vi "Remove Resource.vi"(8 "error in (no error)":errorcluster, 10 "RID":string, 11 "LangFile in":refnum<class "Resource Data.lvclass">) -> (0 "error out":errorcluster, 3 "LangFile out":refnum<class "Resource Data.lvclass">)   [LabVIEW 2013, in "SET Project Data.lvlib" / "Resource Data.lvclass"]
uses:
  Resource Data.lvclass
  Resource Data.lvclass/Resource Data.ctl
  Read Resources.vi
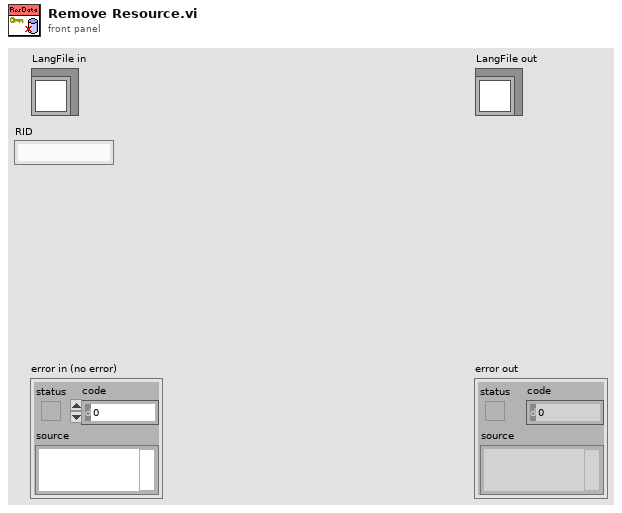
[diagram p1: front panel]
types:
  T1 = typedef "SET Project Data.lvlib/ProjFile_Resource Data.ctl" = cluster{"RID":string, "Tag":string, "Strings [] (UTF-16)":string[], "Shared?":bool}
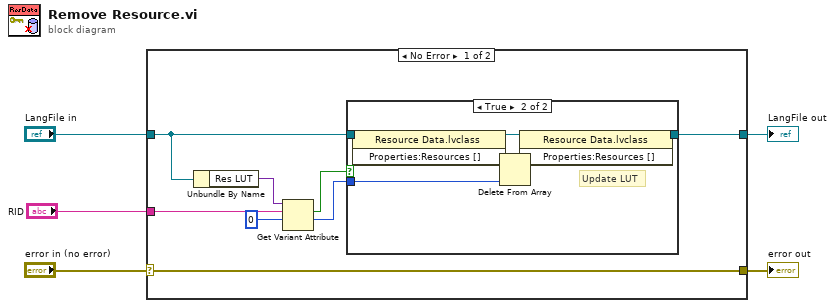
[diagram p0: block diagram]
diagram:
  n1 = case shown="No Error" "error in (no error)" {
    selector: "error in (no error)" -> [w13 w22]
    tunnel: [w13 w22] -> w4
    tunnel: [w6 w21] -> w2
    tunnel: "LangFile in" -> [w7 w21]
    tunnel: "RID" -> [w11 _]
    frame No Error {
      n2 = Unbundle By Name(w7) -> ("Res LUT"=w10:variant)
      n3 = Get Variant Attribute(Variant=w10, name=w11, default value (empty Variant)=0) -> (found=w9:bool, value=w8:i32)  [unwired: 1 in, 2 out]
      n4 = case shown="True" w9 {
        tunnel: w8 -> [_ w20]
        tunnel: w7 -> [w14 w18]
        tunnel: [w14 w19] -> w6
        frame False {
        }
        frame True {
          # "Update LUT"
          n5 = property class="Resource Data.lvclass"(reference=w18) -> (reference out=w15:refnum<class "Resource Data.lvclass">, "Properties:Resources []"=w17:T1[])  [unwired: 1 in, 1 out]
          n6 = Delete From Array(array=w17, index=w20) -> (array with subset deleted=w16:T1[])  [unwired: 1 in, 1 out]
          n7 = property class="Resource Data.lvclass"(reference=w15, "Properties:Resources []"=w16) -> (reference out=w19:refnum<class "Resource Data.lvclass">)  [unwired: 1 in, 1 out]
        }
      }
    }
    frame Error {
    }
  }
  "error out" <- w4
  "LangFile out" <- w2
